vi "GrabImageTest.vi"() -> ()   [LabVIEW 2017]
uses:
  <userlib>/PlayNitrideCameraComponet1010_4/PlayNitrideCameraComponet1010_4.lvlib
panel:
  in  "cameraId":u32
  out "image":T1(plugin-control)
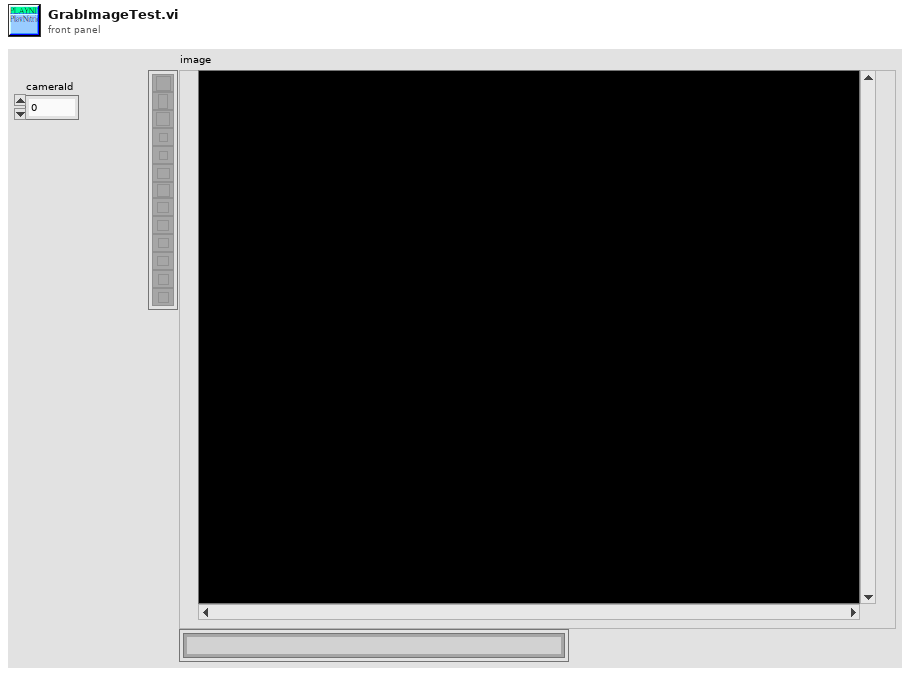
[diagram p1: front panel]
types:
  T1 = typedef "IMAQ Image.ctl" = refnum<image>
  T2 = typedef "Image Type" = u32
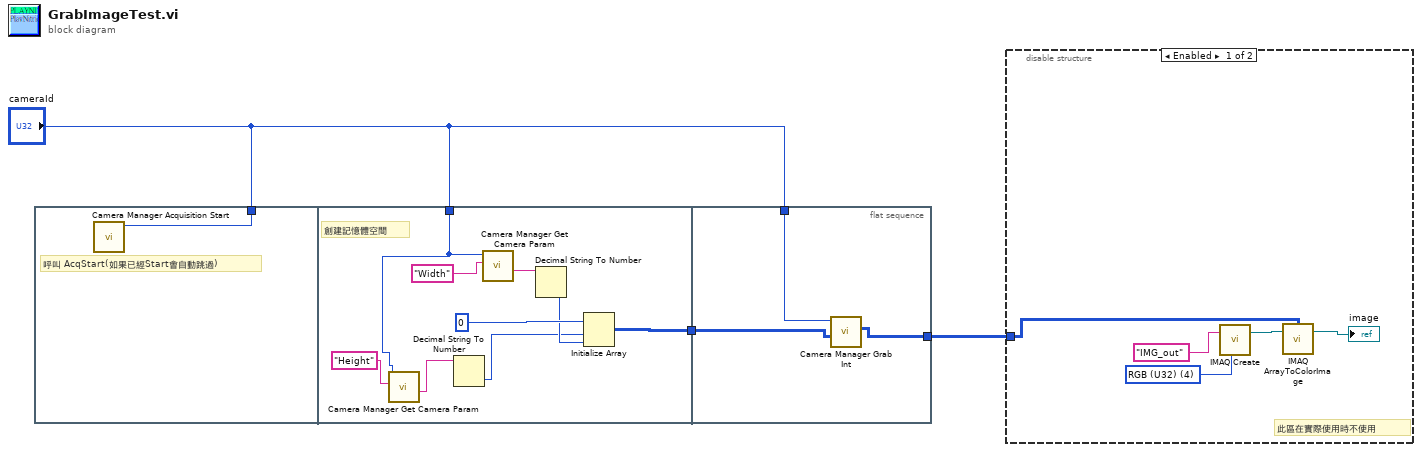
[diagram p0: block diagram]
diagram:
  n1 = flat-sequence {
    tunnel: "cameraId" -> [w4]
    tunnel: [w12] -> w2
    tunnel: "cameraId" -> [w5]
    tunnel: [w14] -> w3
    tunnel: "cameraId" -> [w16]
    tunnel: w2 -> [w15]
    frame #0 {
      # "呼叫 AcqStart(如果已經Start會自動跳過)"
      n2 = call <userlib>:"Camera Manager Acquisition Start.vi"("cameraId"=w4) -> ()  [unwired: 10 in, 1 out]
    }
    frame #1 {
      # "創建記憶體空間"
      n3 = call <userlib>:"Camera Manager Get Camera Param.vi"("NodeName"="Height", "cameraId"=w5) -> ("Value out"=w7:string)  [unwired: 7 in, 2 out]
      n4 = Decimal String To Number(string=w7) -> (number=w10:i32)  [unwired: 2 in, 1 out]
      n5 = call <userlib>:"Camera Manager Get Camera Param.vi"("NodeName"="Width", "cameraId"=w5) -> ("Value out"=w9:string)  [unwired: 7 in, 2 out]
      n6 = Decimal String To Number(string=w9) -> (number=w11:i32)  [unwired: 2 in, 1 out]
      n7 = Initialize Array(u32 0 ("unsigned 32bit integer"), w10, w11) -> (w12:u32[][])
    }
    frame #2 {
      n8 = call <userlib>:"Camera Manager Grab Int.vi"("imgPtr Input"=w15, "cameraId"=w16) -> ("imgPtr"=w14:i32[][])  [unwired: 8 in, 1 out]
    }
  }
  n9 = disable-structure shown="Enabled" {
    disable-tunnel: w3 -> [w17 _]
    frame Enabled {
      w18 = T2 4 items=["Grayscale (U8)", "Grayscale (I16)", "Grayscale (SGL)", "Complex (CSG)", "RGB (U32)", "HSL (U32)", "RGB (U64)", "Grayscale (U16)"] ("Image Type")
      # "此區在實際使用時不使用"
      n10 = call "IMAQ Create"("Image Name"="IMG_out", "Image Type"=w18) -> ("New Image"=w21:T1)  [unwired: 3 in, 1 out]
      n11 = call "IMAQ ArrayToColorImage"("Image Pixels (U32)"=w17, "Image"=w21) -> ("Image Out"=→"image":T1)  [unwired: 3 in, 1 out]
    }
    frame Disabled {
    }
  }
